vi "Generate Signals(SubVI).vi"(10 "Input Parameters":T1, 11 "Sample Index":i32) -> (3 "Data Out":dbl[][](array[numeric]))   [LabVIEW 2012]
doc: "This VI generates a sine wave, white noise and Ramp signals by using parameters entered by the user."
uses:
  <vilib>/Analysis/1siggen.llb/Ramp Pattern by Samples.vi
  <vilib>/Analysis/NI_AALBase.lvlib
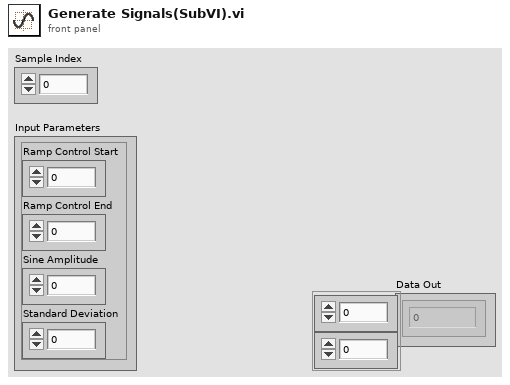
[diagram p1: front panel]
types:
  T1 = cluster{"Ramp Control Start":dbl, "Ramp Control End":dbl, "Sine Amplitude":dbl, "Standard Deviation":dbl}
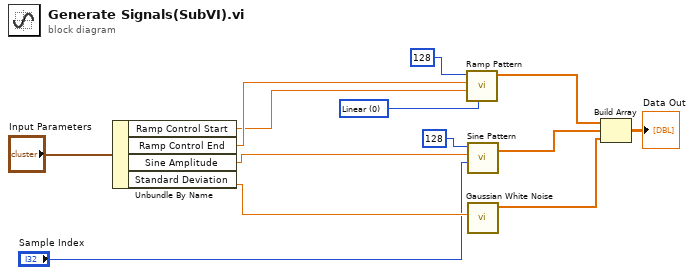
[diagram p0: block diagram]
diagram:
  w2 = u16 0 items=["Linear", "Logarithmic"] ("type")
  n1 = Unbundle By Name("Input Parameters") -> ("Ramp Control Start"=w12:dbl, "Ramp Control End"=w13:dbl, "Sine Amplitude"=w10:dbl, "Standard Deviation"=w9:dbl)
  n2 = call-poly <vilib>:"Ramp Pattern.vi"("type"=w2, "start"=w12, "end"=w13, "samples"=128) -> ("Ramp Pattern"=w4:dbl[])  [unwired: 6 in, 1 out]
  n3 = call <vilib>:"Sine Pattern.vi"("phase(degrees)"="Sample Index", "amplitude"=w10, "samples"=128) -> ("Sinusoidal Pattern"=w5:dbl[])  [unwired: 1 in, 1 out]
  n4 = call <vilib>:"Gaussian White Noise.vi"("standard deviation"=w9) -> ("Gaussian noise pattern"=w6:dbl[])  [unwired: 9 in, 1 out]
  n5 = Build Array(w4, w5, w6) -> (→"Data Out":dbl[][])
